vi "Database Connection.vi"() -> ()   [LabVIEW 2012]
doc: "This example shows three different methods available to connect to a database: \n\n1) An ODBC data source name (DSN) that has been created from the Control Panel with the Data Sources (ODBC) utility. When you installed the LabVIEW Database Tools, a DSN named LabVIEW was automatically created. This LabVIEW DSN uses the Microsoft Access Driver and refers to the database file labview.mdb in the examples\\database directory.\n\n2) A universal data link (UDL) file created from the LabVIEW Tools>>Create Data Link option. When you installed the LabVIEW Database Tools, the LabVIEW.udl file in the examples\\database directory and UDL file extensions were registered in the Windows registry. \n\n3) A dialog prompt can be used to select the data link properties for a database connection."
uses:
  Connection.llb/DB Tools Open Connec (Path).vi
  Connection.llb/DB Tools Open Connec (String).vi
  NI_Database_API_64.lvlib
panel:
  out "Connection Succeeded?":bool
  in  "Connection Method":enum16{"ODBC System DSN", "UDL File", "Prompt"}(ring)
  # "This VI shows three different methods available to connect to a database: an ODBC data source name (DSN), universal data link (UDL) file, or using a dialog prompt."
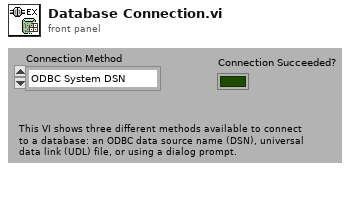
[diagram p1: front panel]
types:
  T1 = typedef "NI_Database_API_64.lvlib/Conn ObjectReference.ctl" = refnum<k1>
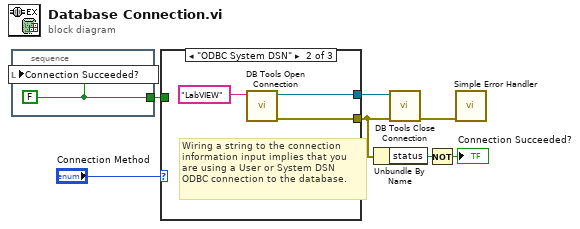
[diagram p0: block diagram]
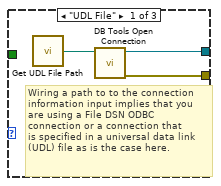
[diagram p2: hidden frame]
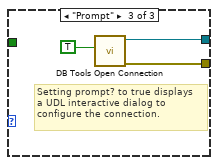
[diagram p3: hidden frame]
diagram:
  n1 = stacked-sequence {
    tunnel: [w8] -> w6
    frame #0 {
      w8 = FALSE ("connection succeeded?")
      n2 = local write "Connection Succeeded?"(w8) -> ()
    }
  }
  n3 = case shown="\"ODBC System DSN\"" "Connection Method" {
    tunnel: [w10 w13 w17] -> w4
    tunnel: [w11 w12 w16] -> w1
    tunnel: w6 -> [_ _ _]
    frame "UDL File" {
      # "Wiring a path to to the connection\ninformation input implies that you \nare using a File DSN ODBC \nconnection or a connection that \nis specified in a universal data link \n(UDL) file as is the case here."
      n4 = call "Get UDL File Path.vi"() -> ("UDL file path"=w9:path)  [unwired: 1 in]
      n5 = call-poly "DB Tools Open Connection.vi"("connection information"=w9) -> ("error out"=w11:errorcluster, "connection reference"=w10:T1)  [unwired: 7 in]
    }
    frame "ODBC System DSN" {
      # "Wiring a string to the connection \ninformation input implies that you \nare using a User or System DSN \nODBC connection to the database."
      n6 = call-poly "DB Tools Open Connection.vi"("connection information"="LabVIEW") -> ("error out"=w12:errorcluster, "connection reference"=w13:T1)  [unwired: 7 in]
    }
    frame "Prompt" {
      # "Setting prompt? to true displays \na UDL interactive dialog to \nconfigure the connection."
      n7 = call-poly "DB Tools Open Connection.vi"("prompt? (F)"=TRUE ("prompt? (f)")) -> ("error out"=w16:errorcluster, "connection reference"=w17:T1)  [unwired: 7 in]
    }
  }
  n8 = Unbundle By Name(w1) -> ("status"=w2:bool)
  n9 = call "DB Tools Close Connection.vi"("error in (no error)"=w1, "connection reference"=w4) -> ("error out"=w5:errorcluster)  [unwired: 5 in]
  n10 = Not(x=w2) -> (.not. x?=→"Connection Succeeded?":bool)
  n11 = call <vilib>:"Simple Error Handler.vi"("error in (no error)"=w5) -> ()  [unwired: 4 in, 5 out]
